vi "Error Process.vi"(8 "error in (no error)":errorcluster, 11 "View Model":T1) -> (0 "error out":errorcluster)   [LabVIEW 2017]
doc: "Error handler provede Error processing depending from it level.\n[Covers: EH1]"
uses:
  View Model/Controls/View Model.ctl
  View Model/Controls/Shared Model.ctl
  Controls/Error Model.ctl
  Controls/Error Message.ctl
  Controls/Error Level.ctl
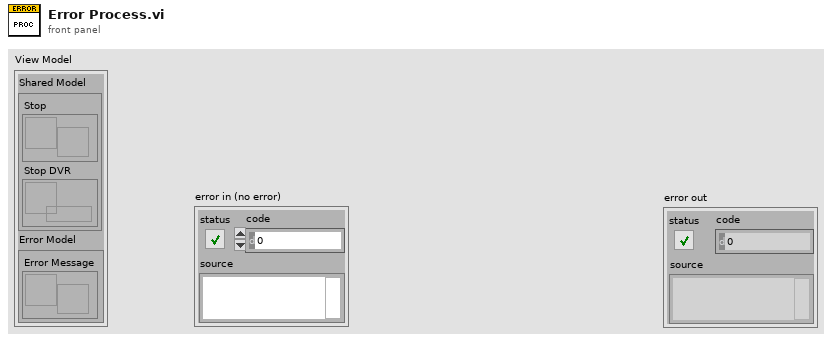
[diagram p1: front panel]
types:
  T1 = typedef "View Model.ctl" = cluster{"Shared Model":T2, "Error Model":T3}
  T2 = typedef "Shared Model.ctl" = cluster{"Stop":refnum<user-event>, "Stop DVR":refnum<data-value>}
  T3 = typedef "Error Model.ctl" = cluster{"Error Message":refnum<user-event>}
  T4 = typedef "Error Level.ctl" = enum16{"Minor Error", "Wash Cycle Error", "System Error"}
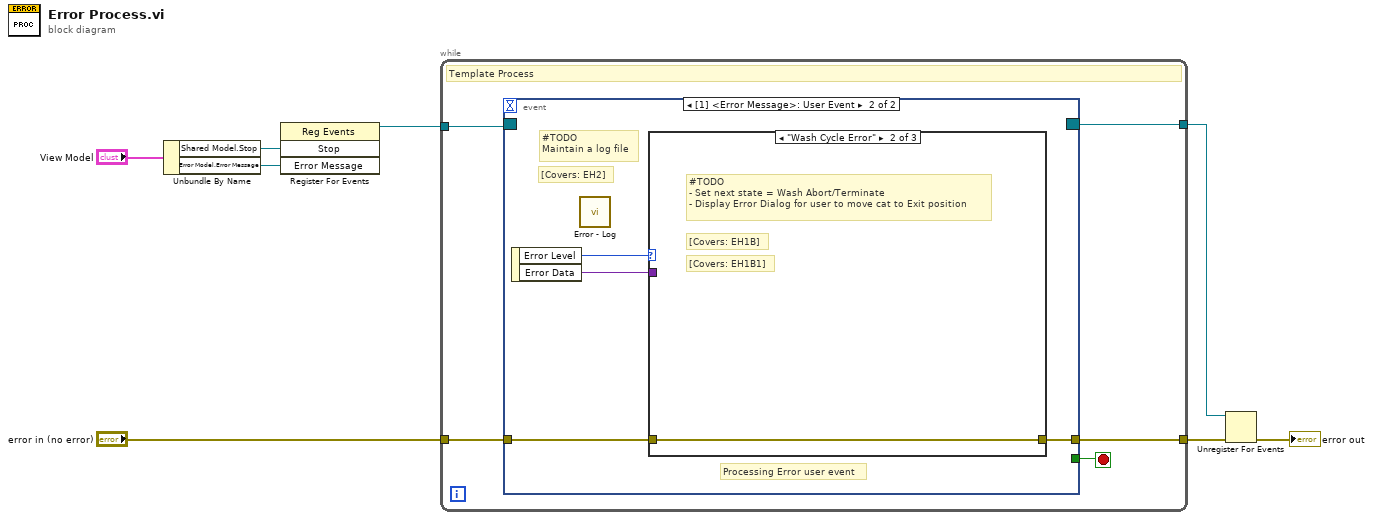
[diagram p0: block diagram]
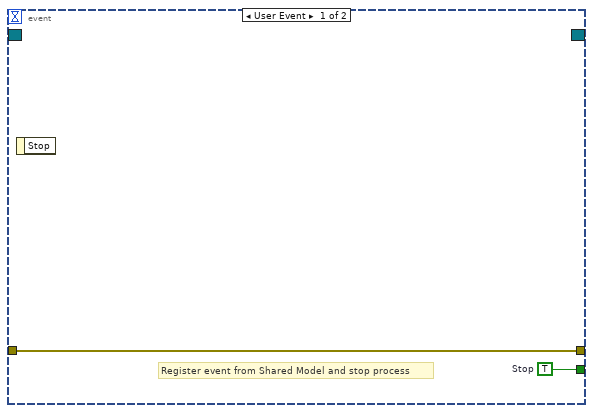
[diagram p2: hidden frame]
diagram:
  n1 = Unbundle By Name("View Model") -> ("Shared Model.Stop"=w7:refnum<user-event>, "Error Model.Error Message"=w1:refnum<user-event>)
  n2 = register-events(w7, w1) -> (reference out=w6:refnum<event-registration>)  [unwired: 2 in, 1 out]
  n3 = while {
    tunnel: w6 -> [w13]
    tunnel: "error in (no error)" -> [w12]
    tunnel: [w11] -> w4
    tunnel: [w9] -> w5
    stop <- w10 stop-if-true
    # "Template Process"
    n4 = event shown="[1] <Error Message>: User Event" {
      selector: w13 -> [_ _]
      dyn-events: [_ _] -> w9
      timeout: _ -> [_ _]
      tunnel: w12 -> [w15 w17]
      tunnel: [w15 w16] -> w11
      tunnel: [w14 _] -> w10
      event User Event {
        w14 = TRUE  # Stop
        # "Register event from Shared Model and stop process"
        n5 = event-data() -> ()  [unwired: 1 in, 1 out]
      }
      event User Event {
        # "[Covers: EH2]"
        # "#TODO\nMaintain a log file"
        # "Processing Error user event"
        n6 = event-data() -> ("Error Level"=w19:T4, "Error Data"=w18:variant)  [unwired: 1 in]
        n7 = call "Error - Log.vi"() -> ()  [unwired: 11 in, 1 out]
        n8 = case shown="\"Wash Cycle Error\"" w19 {
          tunnel: w18 -> [_ _ _]
          tunnel: w17 -> [w20 w21 w22]
          tunnel: [w20 w21 w22] -> w16
          frame "Minor Error", Default {
            # "[Covers: EH1A]"
            # "#TODO\nThis Error invisible for user.\nDo not provide any interruption for operations."
          }
          frame "Wash Cycle Error" {
            # "[Covers: EH1B1]"
            # "[Covers: EH1B]"
            # "#TODO\n- Set next state = Wash Abort/Terminate\n- Display Error Dialog for user to move cat to Exit position"
          }
          frame "System Error" {
            # "[Covers: EH1C3]"
            # "[Covers: EH1C2]"
            # "[Covers: EH1C1]"
            # "[Covers: EH1C]"
            # "#TODO\n- Set next state = Wash Abort/Terminate\n- Display Error Dialog for user to move cat to Exit position\n- Fire Stop User Event for shutdown all consoles, HW, and Terminate application"
          }
        }
      }
    }
  }
  n9 = Unregister For Events(event registration refnum=w5, error in=w4) -> (error out=→"error out":errorcluster)
